vi "Read Display Range Configuration.vi"(8 "error in (no error)":errorcluster, 11 "VGC in":refnum<class "PL Inficon VGC.lvclass">) -> (0 "error out":errorcluster, 2 "mode":u16(ring) items=["UR/OR", "value"], 3 "VGC out":refnum<class "PL Inficon VGC.lvclass">)   [LabVIEW 2015, in "PL Inficon VGC.lvclass"]
doc: "Reads whether UR/OR or value is displayed when an underrange or\noverrange occurs."
uses:
  PL Inficon VGC.lvclass
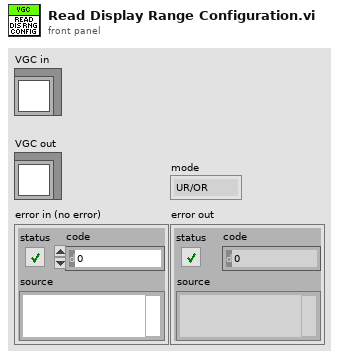
[diagram p1: front panel]
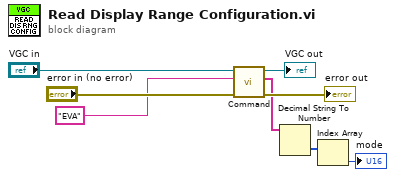
[diagram p0: block diagram]
diagram:
  n1 = call "Command.vi"("error in (no error)"="error in (no error)", "command"="EVA" ("format string"), "VGC in"="VGC in") -> ("error out"=→"error out":errorcluster, "response data"=w3:string[], "VGC out"=→"VGC out":refnum<class "PL Inficon VGC.lvclass">)  [unwired: 6 in]
  n2 = Decimal String To Number(string=w3) -> (number=w4:i32[])  [unwired: 2 in, 1 out]
  n3 = Index Array(array=w4) -> (element=→"mode":i32)  [unwired: 1 in]
